vi "Receive Message.vi"(8 "error in (no error)":errorcluster, 9 "timeout ms (25000)":i32, 10 "bytes to read":i32, 11 "object in":refnum<class "Laser_Ethernet.lvclass">) -> (0 "error out":errorcluster, 2 "Data":string, 3 "object out":refnum<class "Laser_Ethernet.lvclass">)   [LabVIEW 2023, in "Laser_Ethernet.lvclass"]
uses:
  Laser_Ethernet.lvclass
  Laser_Ethernet.lvclass/Laser_Ethernet.ctl
panel:
  out "Checksum OK":bool
  out "Data Size":u32
  out "Execution Code":u16
  out "Answer":u16
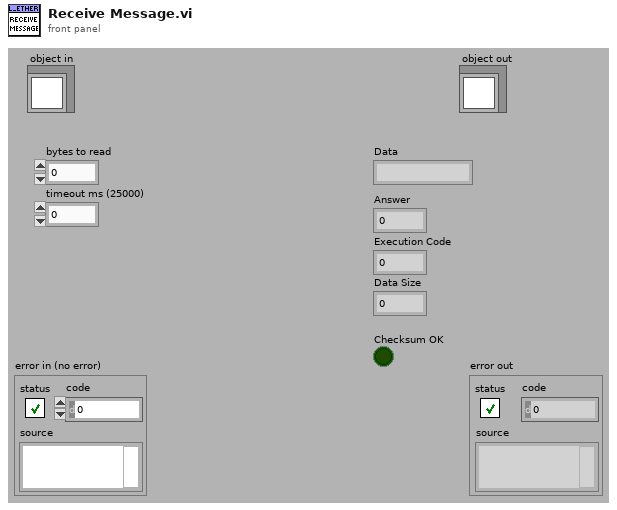
[diagram p1: front panel]
types:
  T1 = enum16{"big-endian, network order", "native, host order", "little-endian"}
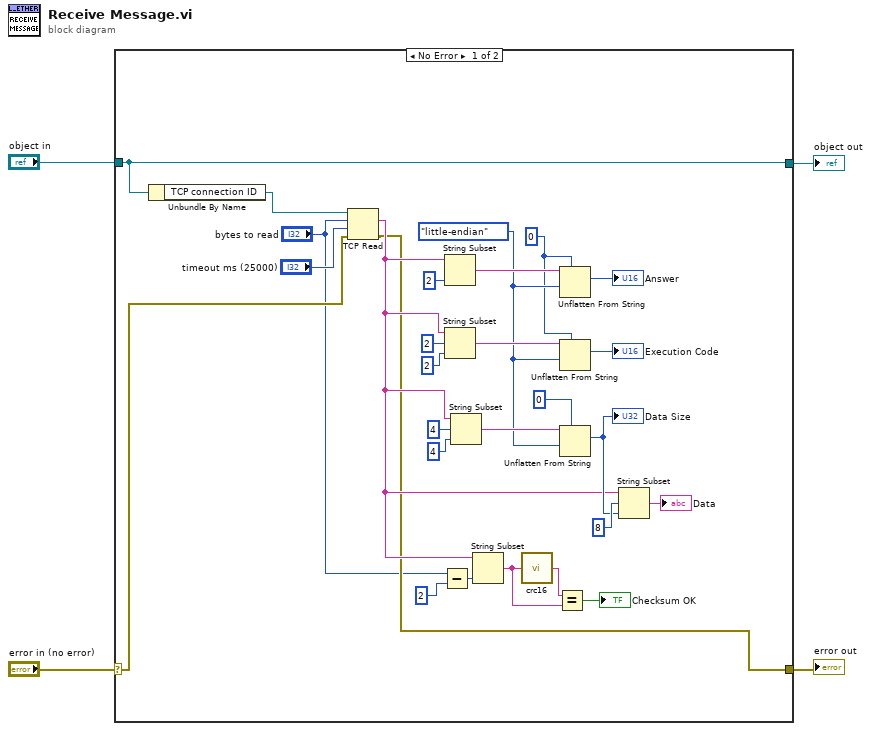
[diagram p0: block diagram]
diagram:
  n1 = case shown="No Error" "error in (no error)" {
    selector: "error in (no error)" -> [w9 w34]
    tunnel: [w8 w34] -> w3
    tunnel: [w11 w33] -> w1
    tunnel: "object in" -> [w11 w33]
    frame No Error {
      w21 = u16 0 ("offset (0)")
      w25 = T1."little-endian" ("byte order (0:big-endian, network order)")
      n2 = Unbundle By Name(w11) -> ("TCP connection ID"=w10:refnum<k5>)
      n3 = TCP Read(connection ID=w10, bytes to read="bytes to read", error in (no error)=w9, 9:"timeout ms (25000)") -> (data out=w12:string, error out=w8:errorcluster)  [unwired: 1 in, 1 out]
      n4 = Subtract(x="bytes to read", y=2) -> (x-y=w14:i32)
      n5 = String Subset(string=w12, length (rest)=2 ("length (rest)")) -> (substring=w30:string)  [unwired: 1 in]
      n6 = String Subset(string=w12, offset (0)=2, length (rest)=2 ("length (rest)")) -> (substring=w29:string)
      n7 = String Subset(string=w12, offset (0)=4, length (rest)=4 ("length (rest)")) -> (substring=w26:string)
      n8 = String Subset(string=w12, length (rest)=w14) -> (substring=w7:string)  [unwired: 1 in]
      n9 = call "crc16.vi"("Message"=w7) -> ("crc 16"=w6:string)
      n10 = Equal?(x=w6, y=w7) -> (x = y?=→"Checksum OK":bool)
      n11 = Unflatten From String(type=w21, binary string=w30, byte order (0:big-endian, network order)=w25) -> (value=→"Answer":u16)  [unwired: 2 in, 2 out]
      n12 = Unflatten From String(type=w21, binary string=w29, byte order (0:big-endian, network order)=w25) -> (value=→"Execution Code":u16)  [unwired: 2 in, 2 out]
      n13 = Unflatten From String(type=u32 0 ("offset (0)"), binary string=w26, byte order (0:big-endian, network order)=w25) -> (value=w19:u32)  [unwired: 2 in, 2 out]
      "Data Size" <- w19
      n14 = String Subset(string=w12, offset (0)=8, length (rest)=w19) -> (substring=→"Data":string)
    }
    frame Error {
    }
  }
  "error out" <- w3
  "object out" <- w1
